vi "ServoToZero.vi"(10 "动作IO":enum16{"俯仰轴归0", "旋转轴归0", "空"}(ring)) -> ()   [LabVIEW 2018]
panel:
  out "元素":u16
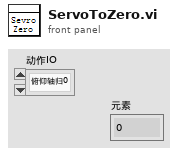
[diagram p1: front panel]
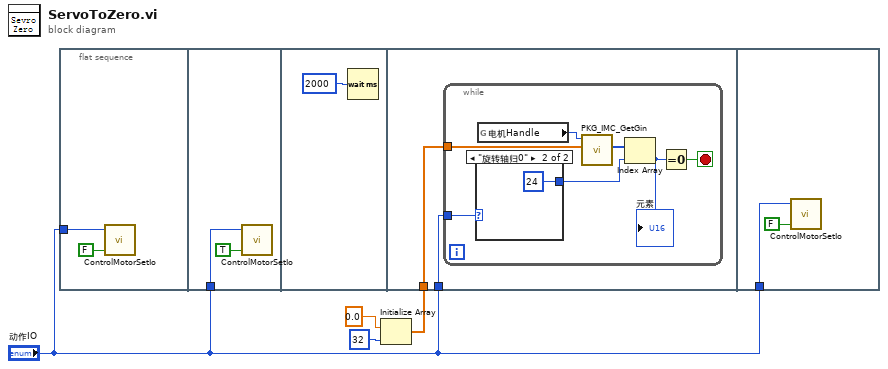
[diagram p0: block diagram]
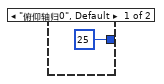
[diagram p2: hidden frame]
diagram:
  n1 = flat-sequence {
    tunnel: "动作IO" -> [w5]
    tunnel: "动作IO" -> [w7]
    tunnel: "动作IO" -> [w11]
    tunnel: w3 -> [w10]
    tunnel: "动作IO" -> [w21]
    frame #0 {
      n2 = call "ControlMotorSetIo.vi"("状态"=FALSE, "动作IO"=w5) -> ()  [unwired: 3 in, 1 out]
    }
    frame #1 {
      n3 = call "ControlMotorSetIo.vi"("状态"=TRUE, "动作IO"=w7) -> ()  [unwired: 3 in, 1 out]
    }
    frame #2 {
      n4 = Wait (ms)(milliseconds to wait=u32 2000 ("等待时间（毫秒）")) -> ()  [unwired: 1 out]
    }
    frame #3 {
      n5 = while {
        tunnel: w11 -> [w17]
        tunnel: w10 -> [w14]
        stop <- w12 stop-if-true
        n6 = case shown="\"旋转轴归0\"" w17 {
          tunnel: [25 24] -> w15
          frame "俯仰轴归0", Default {
          }
          frame "旋转轴归0" {
          }
        }
        n7 = global read "参数.vi" "电机Handle"() -> (w18:u32)
        n8 = call "PKG_IMC_GetGin.vi"("gin"=w14, "Handle"=w18) -> ("gin out"=w16:u16[])  [unwired: 7 in, 2 out]
        n9 = Index Array(array=w16, index=w15) -> (element=w13:u16)
        "元素" <- w13
        n10 = Equal To 0?(x=w13) -> (x = 0?=w12:bool)
      }
    }
    frame #4 {
      n11 = call "ControlMotorSetIo.vi"("状态"=FALSE, "动作IO"=w21) -> ()  [unwired: 3 in, 1 out]
    }
  }
  n12 = Initialize Array(0.0 ("元素"), 32 ("维数大小")) -> (w3:dbl[])
